vi "motor02.vi"() -> ()   [LabVIEW 2019]
uses:
  <vilib>/Platform/TimedLoop/XDataNode/timing_clust.ctl
  <vilib>/Platform/TimedLoop/XDataNode/nitl_modes.ctl
  <vilib>/Platform/TimedLoop/XDataNode/wakeup.ctl
  <vilib>/addons/control/pid/pid.llb/PID (DBL).vi
  <vilib>/platform/TimedLoop/XDataNode/XDataNode.xnode
  <vilib>/addons/control/pid/NI_PID_pid.lvlib
  <vilib>/Platform/TimedLoop/XDataNode/XDNodeRunTimeDep.lvlib
panel:
  in  "stop":bool
  in  "Enum":enum16{"M1", "M2", "M3"}(ring)
  in  "error in (no error)":errorcluster
  in  "Reset":bool
  in  "dt(s)":dbl
  in  "RPM":dbl
  out "error out":errorcluster
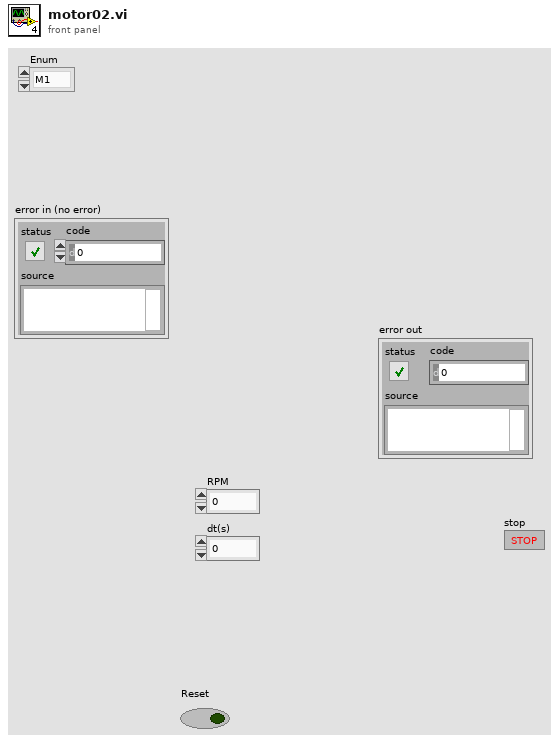
[diagram p1: front panel]
types:
  T1 = typedef "XDNodeRunTimeDep.lvlib/timing_clust.ctl" = cluster{"Expected End [f-1]":u64, "Actual End [f-1]":u64, "Finished Late? [f-1]":bool, "Expected End [i-1]":u64, "Actual End [i-1]":u64, "Finished Late? [i-1]":bool, "Expected Start [i]":u64, "Actual Start [i]":u64, "Expected Start [f]":u64, "Actual Start [f]":u64, "Source Name":string, "Structure Name":string, "Period":i64, "Deadline":i64, "Offset":i64, "Start":i64, "Priority":i32, "Timeout":i32, "Mode":T2, "Wakeup Reason":T3, "Error":errorcluster, "Source Type":string, "Secondary Source Type":string, "Global End Time":u64, "Global Start Time":u64, "Frame Duration":u64, "Iteration Duration":u64, "Assigned CPU":i32, "I/O Scan Engine Mode":u32}
  T2 = typedef "XDNodeRunTimeDep.lvlib/nitl_modes.ctl" = enum32{"No Change", "Process missed periods, maintain original phase", "Discard missed periods, maintain original phase", "Process missed periods, ignore original phase", "Discard missed periods, ignore original phase"}
  T3 = typedef "XDNodeRunTimeDep.lvlib/wakeup.ctl" = enum32{"Normal", "Aborted", "Asynchronous wakeup", "Timing source error", "Timed loop error", "Timeout"}
  T4 = cluster{"proportional gain (Kc)":dbl, "integral time (Ti, min)":dbl, "derivative time (Td, min)":dbl}
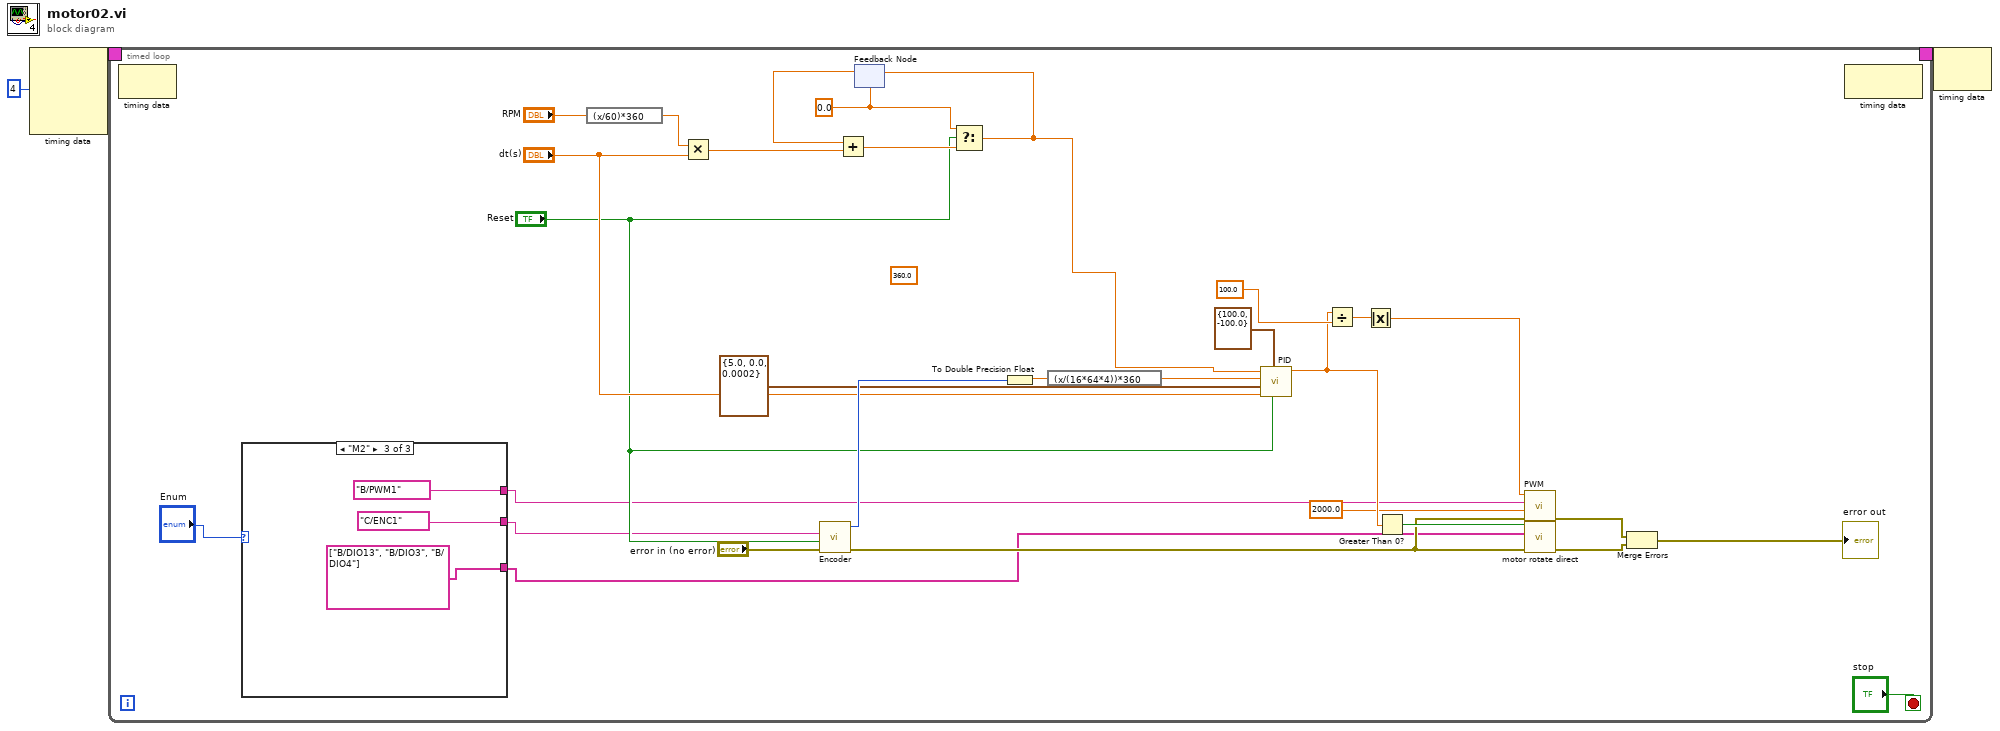
[diagram p0: block diagram]
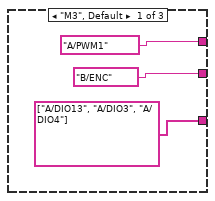
[diagram p2: hidden frame]
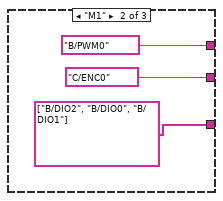
[diagram p3: hidden frame]
diagram:
  n1 = node-c288(i64 4 ("Period")) -> (w3:T1)  [unwired: 3 in]
  n2 = timed-loop {
    timing: w3 -> [_]
    timing-out: [_] -> w2
    stop <- "stop" stop-if-true
    (unwired) 360.0 ("setpoint")
    w21 = 0.0
    n3 = node-c288() -> ()  [unwired: 1 in, 1 out]
    n4 = case shown="\"M2\"" "Enum" {
      tunnel: [tag "B/ENC" ("Channel Name") tag "C/ENC0" ("Channel Name") tag "C/ENC1" ("Channel Name")] -> w6
      tunnel: [tag[] ["A/DIO13", "A/DIO3", "A/DIO4"] ("Channel Names") tag[] ["B/DIO2", "B/DIO0", "B/DIO1"] ("Channel Names") tag[] ["B/DIO13", "B/DIO3", "B/DIO4"] ("Channel Names")] -> w5
      tunnel: [tag "A/PWM1" ("Channel Name") tag "B/PWM0" ("Channel Name") tag "B/PWM1" ("Channel Name")] -> w7
      frame "M3", Default {
      }
      frame "M1" {
      }
      frame "M2" {
      }
    }
    n5 = expression code="(x/60)*360"("RPM") -> (w31:dbl)
    n6 = Multiply(x=w31, y="dt(s)") -> (x*y=w30:dbl)
    n7 = call "Encoder.vi"("error in (no error)"="error in (no error)", "Reset Counter"="Reset", "Channel Name"=w6) -> ("error out"=w14:errorcluster, "Counter Value"=w28:i32)  [unwired: 6 in, 1 out]
    n8 = feedback #1(w21) -> (w29:dbl)
    n9 = Add(x=w29, y=w30) -> (x+y=w22:dbl)
    n10 = Select(t=w21, s="Reset", f=w22) -> (s? t:f=w8:dbl)
    n11 = feedback-in #1(w8) -> ()
    n12 = To Double Precision Float(number=w28) -> (double precision float=w27:dbl)
    n13 = expression code="(x/(16*64*4))*360"(w27) -> (w26:dbl)
    n14 = call-poly <vilib>:"PID.vi"("reinitialize? (F)"="Reset", "output range"=cluster{"output high":dbl, "output low":dbl} {"output high"=100.0, "output low"=-100.0}, "dt (s)"="dt(s)", "PID gains"=T4 {"proportional gain (Kc)"=5.0, "integral time (Ti, min)"=0.0, "derivative time (Td, min)"=0.0002}, "process variable"=w26, "setpoint"=w8) -> ("output"=w17:dbl)  [unwired: 4 in, 1 out]
    n15 = Divide(x=w17, y=100.0 ("output high")) -> (x/y=w19:dbl)
    n16 = Absolute Value(x=w19) -> (abs(x)=w18:dbl)
    n17 = Greater Than 0?(x=w17) -> (x > 0?=w16:bool)
    n18 = call "PWM.vi"("error in (no error)"=w14, "Frequency [Hz]"=2000.0, "Channel Name"=w7, "Duty Cycle"=w18) -> ("error out"=w11:errorcluster)  [unwired: 7 in]
    n19 = call "motor rotate direct.vi"("error in (no error)"=w14, "Channel Names"=w5, "Boolean"=w16) -> ("error out"=w12:errorcluster)  [unwired: 8 in]
    n20 = Merge Errors(w11, w12) -> (→"error out":errorcluster)
    n21 = node-c288() -> ()  [unwired: 1 in, 1 out]
  }
  n22 = node-c288(w2) -> ()  [unwired: 1 out]
